vi "RotateWallSkillVSS.vi"(8 "error in (no error)":errorcluster, 9 "Game":refnum<class "Game.lvclass">, 10 "Robot":refnum<class "Robot.lvclass">, 11 "RotateWallSkillVSS in":refnum<class "RotateWallSkillVSS.lvclass">) -> (0 "error out":errorcluster, 2 "Robot out":refnum<class "Robot.lvclass">, 3 "RotateWallSkillVSS out":refnum<class "RotateWallSkillVSS.lvclass">)   [LabVIEW 2020, in "RotateWallSkillVSS.lvclass"]
uses:
  RotateWallSkillVSS.lvclass
  Robot_class/Robot.lvclass
  C:/Users/lucio/Desktop/Horie/ROBOIME/VSS_AI/Object_class/Object.lvclass
  Game_class/Game.lvclass
  Object_class/Object.lvclass/Object.ctl
  Game_class/Game.lvclass/Game.ctl
  Game_class/Navigation/VSSNavigation/VSSAttackerStates.ctl
  Game_class/Read BallRef.vi
  Game_class/Read FieldRef.vi
  Object_class/Read x.vi
  Object_class/Read y.vi
  Ball_class/Ball.lvclass
  Field_class/Field.lvclass
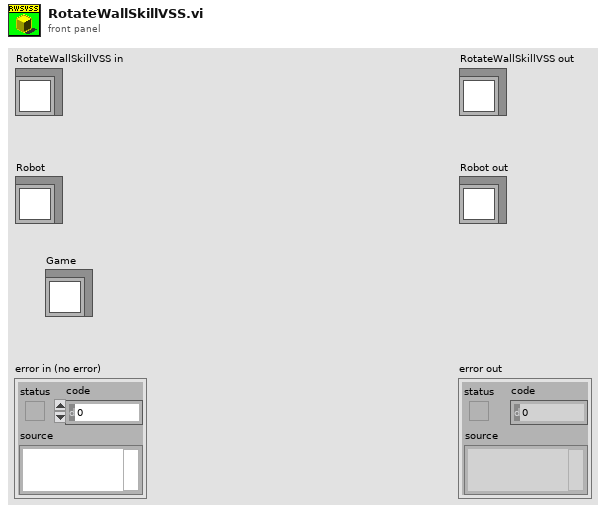
[diagram p1: front panel]
types:
  T1 = typedef "VSSAttackerStates.ctl" = enum16{"Pass", "GoToTangent", "BallGetting", "GoToKick", "Rotate anti-clockwise", "Rotate Clockwise", ""}
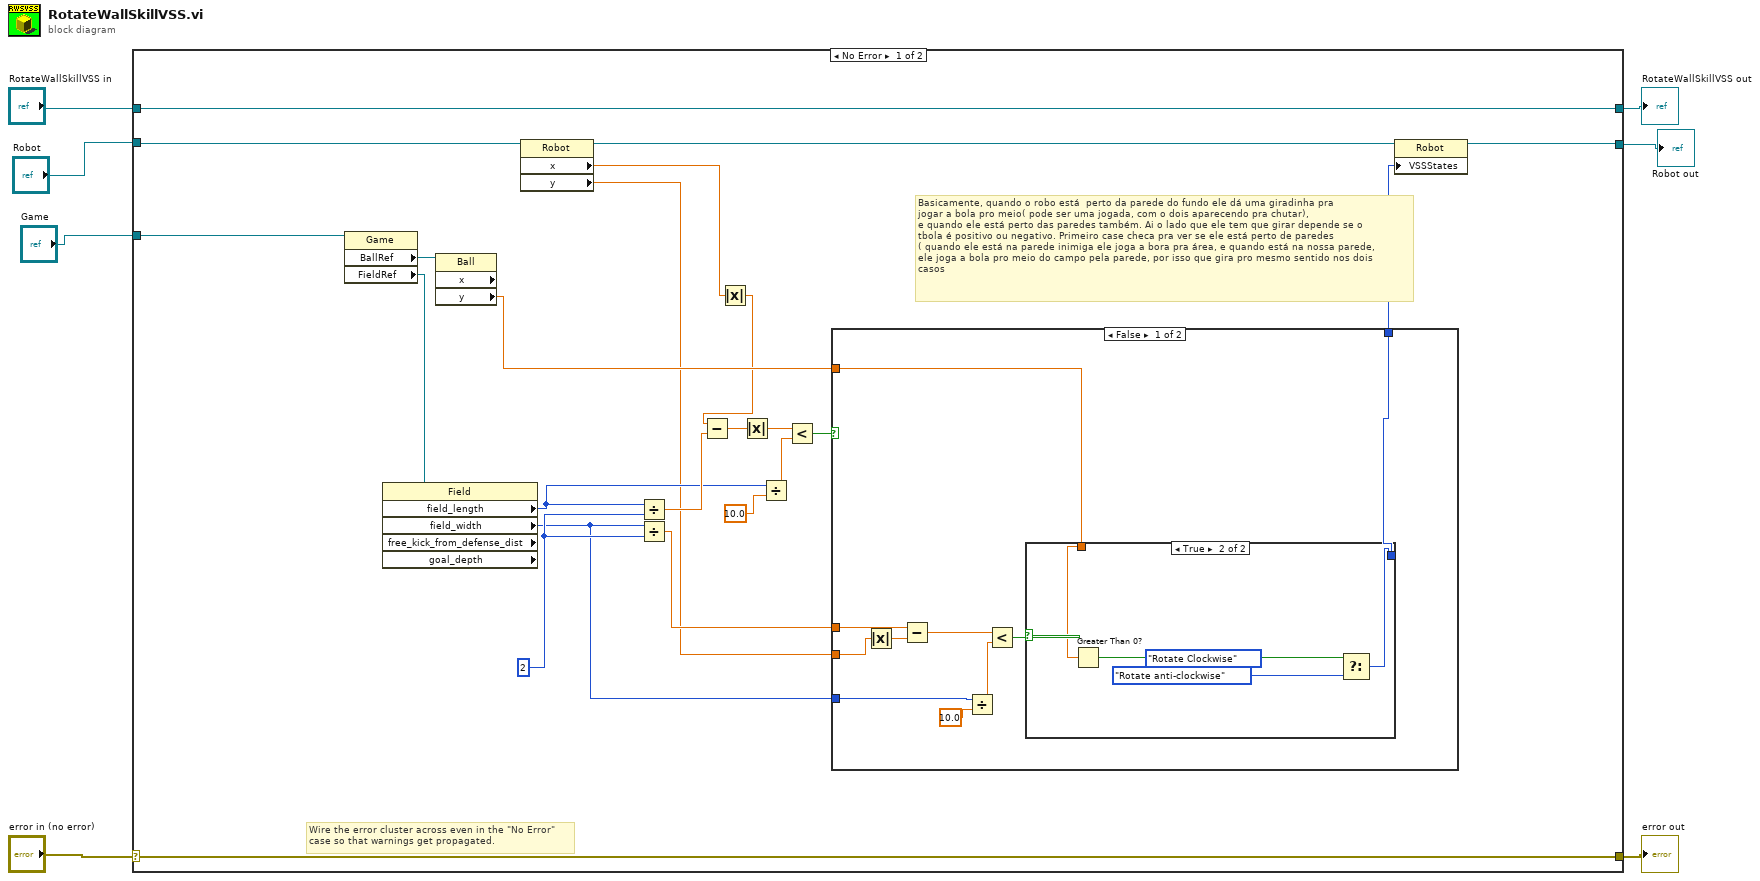
[diagram p0: block diagram]
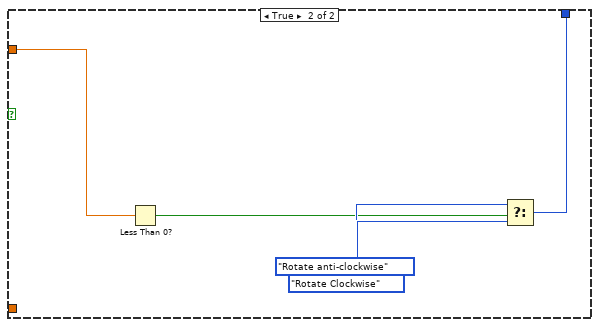
[diagram p3: hidden frame]
diagram:
  n1 = case shown="No Error" "error in (no error)" {
    selector: "error in (no error)" -> [w29 w53]
    tunnel: [w29 w53] -> w6
    tunnel: [w30 w52] -> w4
    tunnel: "RotateWallSkillVSS in" -> [w30 w52]
    tunnel: [w28 w51] -> w3
    tunnel: "Robot" -> [w26 w51]
    tunnel: "Game" -> [w27 _]
    frame No Error {
      w22 = 2
      # "Basicamente, quando o robo está  perto da parede do fundo ele dá uma giradinha pra\njogar a bola pro meio( pode ser uma jogada, com o dois aparecendo pra chutar), \ne quando ele está perto das paredes também. Ai o lado que ele tem que girar depende se o\ntbola é positivo ou negativo. Primeiro case checa pra ver se ele está perto de paredes\n( quando ele está na parede inimiga ele joga a bora pra área, e quando está na nossa parede,\nele joga a bola pro meio do campo pela parede, por isso que gira pro mesmo sentido nos dois\ncasos"
      # "Wire the error cluster across even in the \"No Error\"\ncase so that warnings get propagated."
      n2 = property class="Game"(reference=w27) -> ("BallRef"=w23:refnum<class "Ball.lvclass">, "FieldRef"=w24:refnum<class "Field.lvclass">)  [unwired: 1 in, 2 out]
      n3 = property class="Field" props=["field_length", "field_width", "free_kick_from_defense_dist", "goal_depth"](reference=w24) -> ("field_length"=w16:i32, "field_width"=w12:i32)  [unwired: 1 in, 4 out]
      n4 = property class="Ball" props=["x", "y"](reference=w23) -> ("y"=w13:dbl)  [unwired: 1 in, 3 out]
      n5 = property class="Robot"(reference=w26) -> (reference out=w25:refnum<class "Robot.lvclass">, "x"=w9:dbl, "y"=w10:dbl)  [unwired: 1 in, 1 out]
      n6 = Divide(x=w16, y=w22) -> (x/y=w21:dbl)
      n7 = Divide(x=w12, y=w22) -> (x/y=w11:dbl)
      n8 = Absolute Value(x=w9) -> (abs(x)=w8:dbl)
      n9 = Subtract(x=w8, y=w21) -> (x-y=w20:dbl)
      n10 = Absolute Value(x=w20) -> (abs(x)=w19:dbl)
      n11 = Divide(x=w16, y=10.0) -> (x/y=w17:dbl)
      n12 = Less?(x=w19, y=w17) -> (x < y?=w15:bool)
      n13 = case shown="False" w15 {
        tunnel: [w35 w48] -> w14
        tunnel: w13 -> [w36 w47]
        tunnel: w12 -> [w38 _]
        tunnel: w11 -> [w33 _]
        tunnel: w10 -> [w32 _]
        frame False {
          n14 = Absolute Value(x=w32) -> (abs(x)=w31:dbl)
          n15 = Subtract(x=w33, y=w31) -> (x-y=w34:dbl)
          n16 = Divide(x=w38, y=10.0) -> (x/y=w39:dbl)
          n17 = Less?(x=w34, y=w39) -> (x < y?=w37:bool)
          n18 = case shown="True" w37 {
            tunnel: w36 -> [_ w44]
            tunnel: [_ w41] -> w35
            frame False {
            }
            frame True {
              n19 = Greater Than 0?(x=w44) -> (x > 0?=w45:bool)
              n20 = Select(t=VSSAttackerStates."Rotate Clockwise" ("VSSStates"), s=w45, f=VSSAttackerStates."Rotate anti-clockwise" ("VSSStates")) -> (s? t:f=w41:T1)
            }
          }
        }
        frame True {
          n21 = Less Than 0?(x=w47) -> (x < 0?=w46:bool)
          n22 = Select(t=VSSAttackerStates."Rotate anti-clockwise" ("VSSStates"), s=w46, f=VSSAttackerStates."Rotate Clockwise" ("VSSStates")) -> (s? t:f=w48:T1)
        }
      }
      n23 = property class="Robot"(reference=w25, "VSSStates"=w14) -> (reference out=w28:refnum<class "Robot.lvclass">)  [unwired: 1 in, 1 out]
    }
    frame Error {
    }
  }
  "error out" <- w6
  "RotateWallSkillVSS out" <- w4
  "Robot out" <- w3
